vi "tcp_conn.vi"() -> ()   [LabVIEW 2015]
panel:
  in  "服务器端口":string="7099"
  in  "服务器IP":string="172.20.11.30"
  out "kormee_upload_connid":refnum<k5>
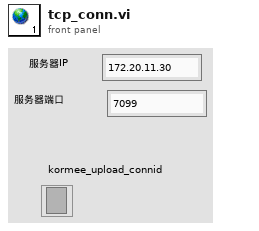
[diagram p1: front panel]
diagram:
